vi "Read Data Titles.vi"(8 "error in (no error)":errorcluster, 11 "ITC 503 in":refnum<class "ITC 503.lvclass">) -> (0 "error out":errorcluster, 2 "Data titles":string[](array[string])=["ITC_T (K)"], 3 "ITC 503 out":refnum<class "ITC 503.lvclass">)   [LabVIEW 2015, in "ITC 503.lvclass"]
uses:
  ITC 503.lvclass
  Controls/ITC503 FP Data.ctl
  OO Devices/Device/Read Controls Snapshot.vi
  OO Devices/Device/Read Control Panel Loaded.vi
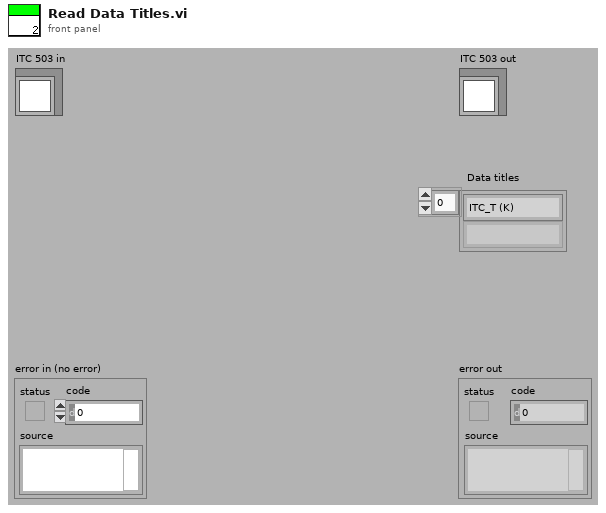
[diagram p1: front panel]
types:
  T1 = typedef "ITC503 FP Data.ctl" = cluster{"Channels to measure":i32[]}
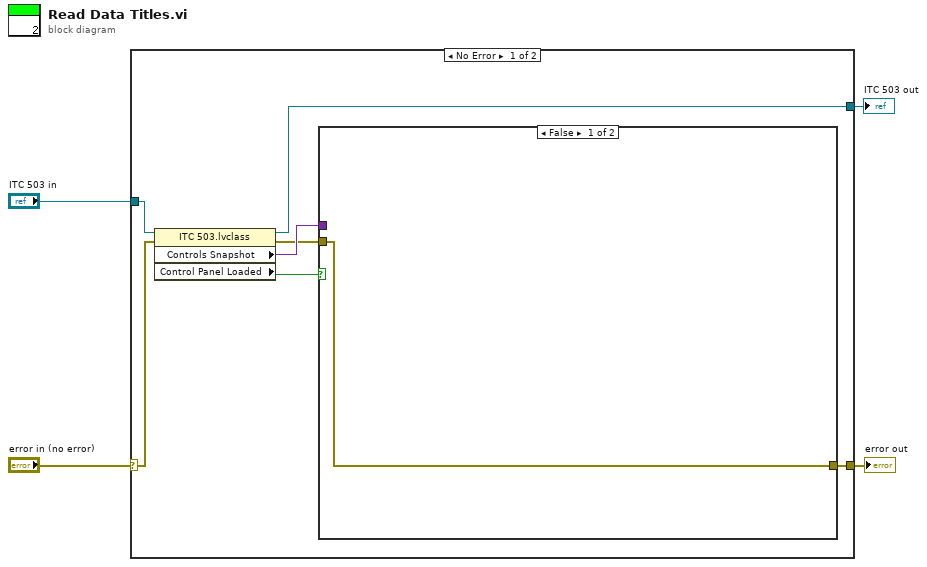
[diagram p0: block diagram]
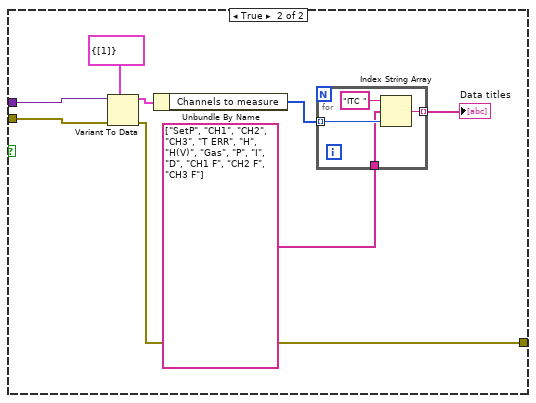
[diagram p2: hidden frame]
diagram:
  n1 = case shown="No Error" "error in (no error)" {
    selector: "error in (no error)" -> [w8 w26]
    tunnel: [w6 w26] -> w3
    tunnel: [w10 w25] -> w1
    tunnel: "ITC 503 in" -> [w11 w25]
    frame No Error {
      n2 = property class="ITC 503.lvclass"(reference=w11, error in=w8) -> (reference out=w10:refnum<class "ITC 503.lvclass">, error out=w7:errorcluster, "Controls Snapshot"=w9:variant, "Control Panel Loaded"=w5:bool)
      n3 = case shown="False" w5 {
        tunnel: w9 -> [_ w20]
        tunnel: w7 -> [w12 w19]
        tunnel: [w12 w13] -> w6
        frame False {
        }
        frame True {
          n4 = Variant To Data(error in=w19, type=T1 {"Channels to measure"=[1]} ("Data"), Variant=w20) -> (data=w17:T1, error out=w13:errorcluster)
          n5 = Unbundle By Name(w17) -> ("Channels to measure"=w16:i32[])
          n6 = for {
            tunnel: w16 -> [w23] mode=indexing
            tunnel: string[] ["SetP", "CH1", "CH2", "CH3", "T ERR", "H", "H(V)", "Gas", "P", "I", "D", "CH1 F", "CH2 F", "CH3 F"] -> [w22]
            tunnel: [w21] -> w14 mode=indexing
            n7 = Index String Array(1:w23, 2:w22, 3:"ITC " ("string (\"\")")) -> (0:w21:string)
          }
          "Data titles" <- w14
        }
      }
    }
    frame Error {
    }
  }
  "error out" <- w3
  "ITC 503 out" <- w1
